vi "Vision Processing.vi"(4 "error in (no error)":errorcluster, 7 "Image Size":T1=enum."320x240") -> ()   [LabVIEW 2015]
doc: "This VI runs in parallel to other tasks. It gets images from the camera, processes them for color or shape and use that information to affect robot behavior."
uses:
  <vilib>/Rock Robotics/WPI/Camera/WPI_CameraImageSize.ctl
  <vilib>/Rock Robotics/WPI/Camera/WPI_CameraWhite Balance Values.ctl
  <vilib>/Rock Robotics/WPI/Camera/WPI_CameraExposure Values.ctl
  <vilib>/Rock Robotics/WPI/Camera/WPI_CameraFrameRate.ctl
  Robot Global Data.vi
panel:
  in  "Image Size 2":T1=enum."320x240"
  in  "error in (no error) 2":errorcluster
  in  "stop":bool
  in  "Target Template":enum32{"Template 3", "Template 1", "Template 2"}(radio)=enum."Template 1"
  out "Input Image":T2(plugin-control)
  out "Processed Image":T2(plugin-control)
  in  "Loop Delay (ms)":u32(slide)=200 scale=0.0..250.0
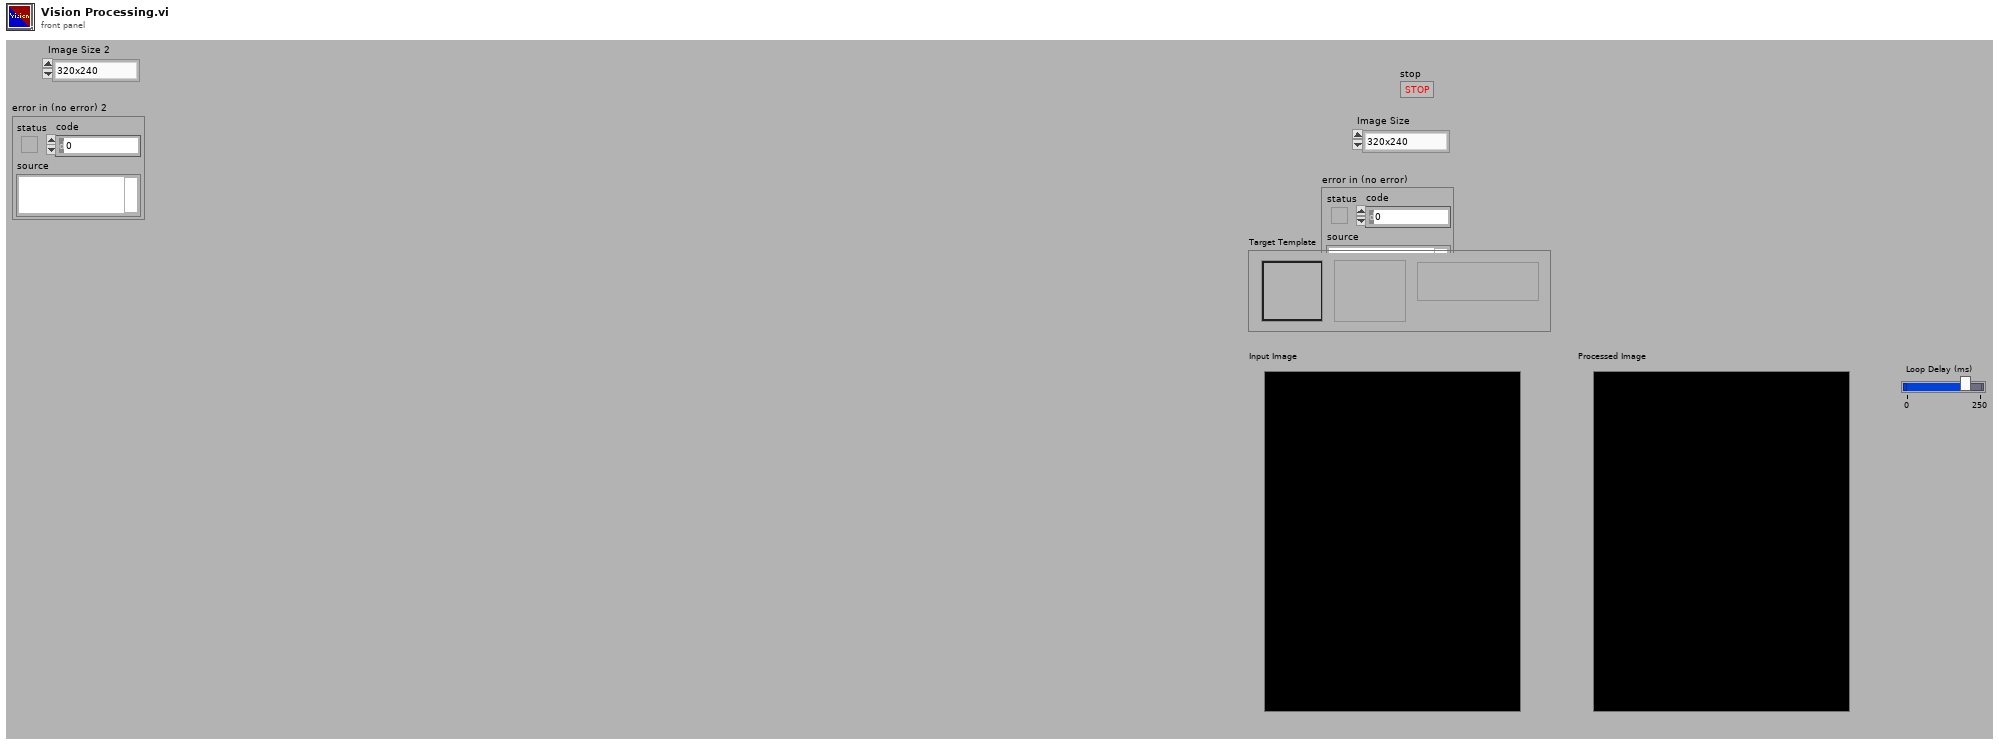
[diagram p1: front panel]
types:
  T1 = typedef "WPI_CameraImageSize.ctl" = enum16{"640x480", "320x240", "160x120", "Custom"}
  T2 = typedef "IMAQ Image.ctl" = refnum<image>
  T3 = typedef "WPI_CameraFrameRate.ctl" = u32
  T4 = typedef "WPI_CameraExposure Values.ctl" = enum16{"Auto", "Flicker-free 50 Hz", "Flicker-free 60 Hz", "Hold current", "Custom"}
  T5 = typedef "WPI_CameraWhite Balance Values.ctl" = enum16{"Auto", "Fixed indoor", "Fixed outdoor 1", "Fixed outdoor 2", "Fixed fluorescent 1", "Fixed fluorescent 2", "Hold current", "Custom"}
  T6 = typedef "Image Type" = u32
  T7 = typedef "WPI_CameraDevRef.ctl" = cluster{"Camera Address":string, "CameraStatus":errorcluster}
  T8 = cluster{"Position":cluster{"x":sgl, "y":sgl}, "Angle":sgl, "Scale":sgl, "Score":sgl, "Bounding Box":cluster{"x":sgl, "y":sgl}[]}[]
  T9 = typedef "ROI Descriptor" = cluster{"Global Rectangle":i32[], "Contours":cluster{"ID":enum32{"External", "Internal"}, "Type":u32, "Coordinates":i32[]}[]}
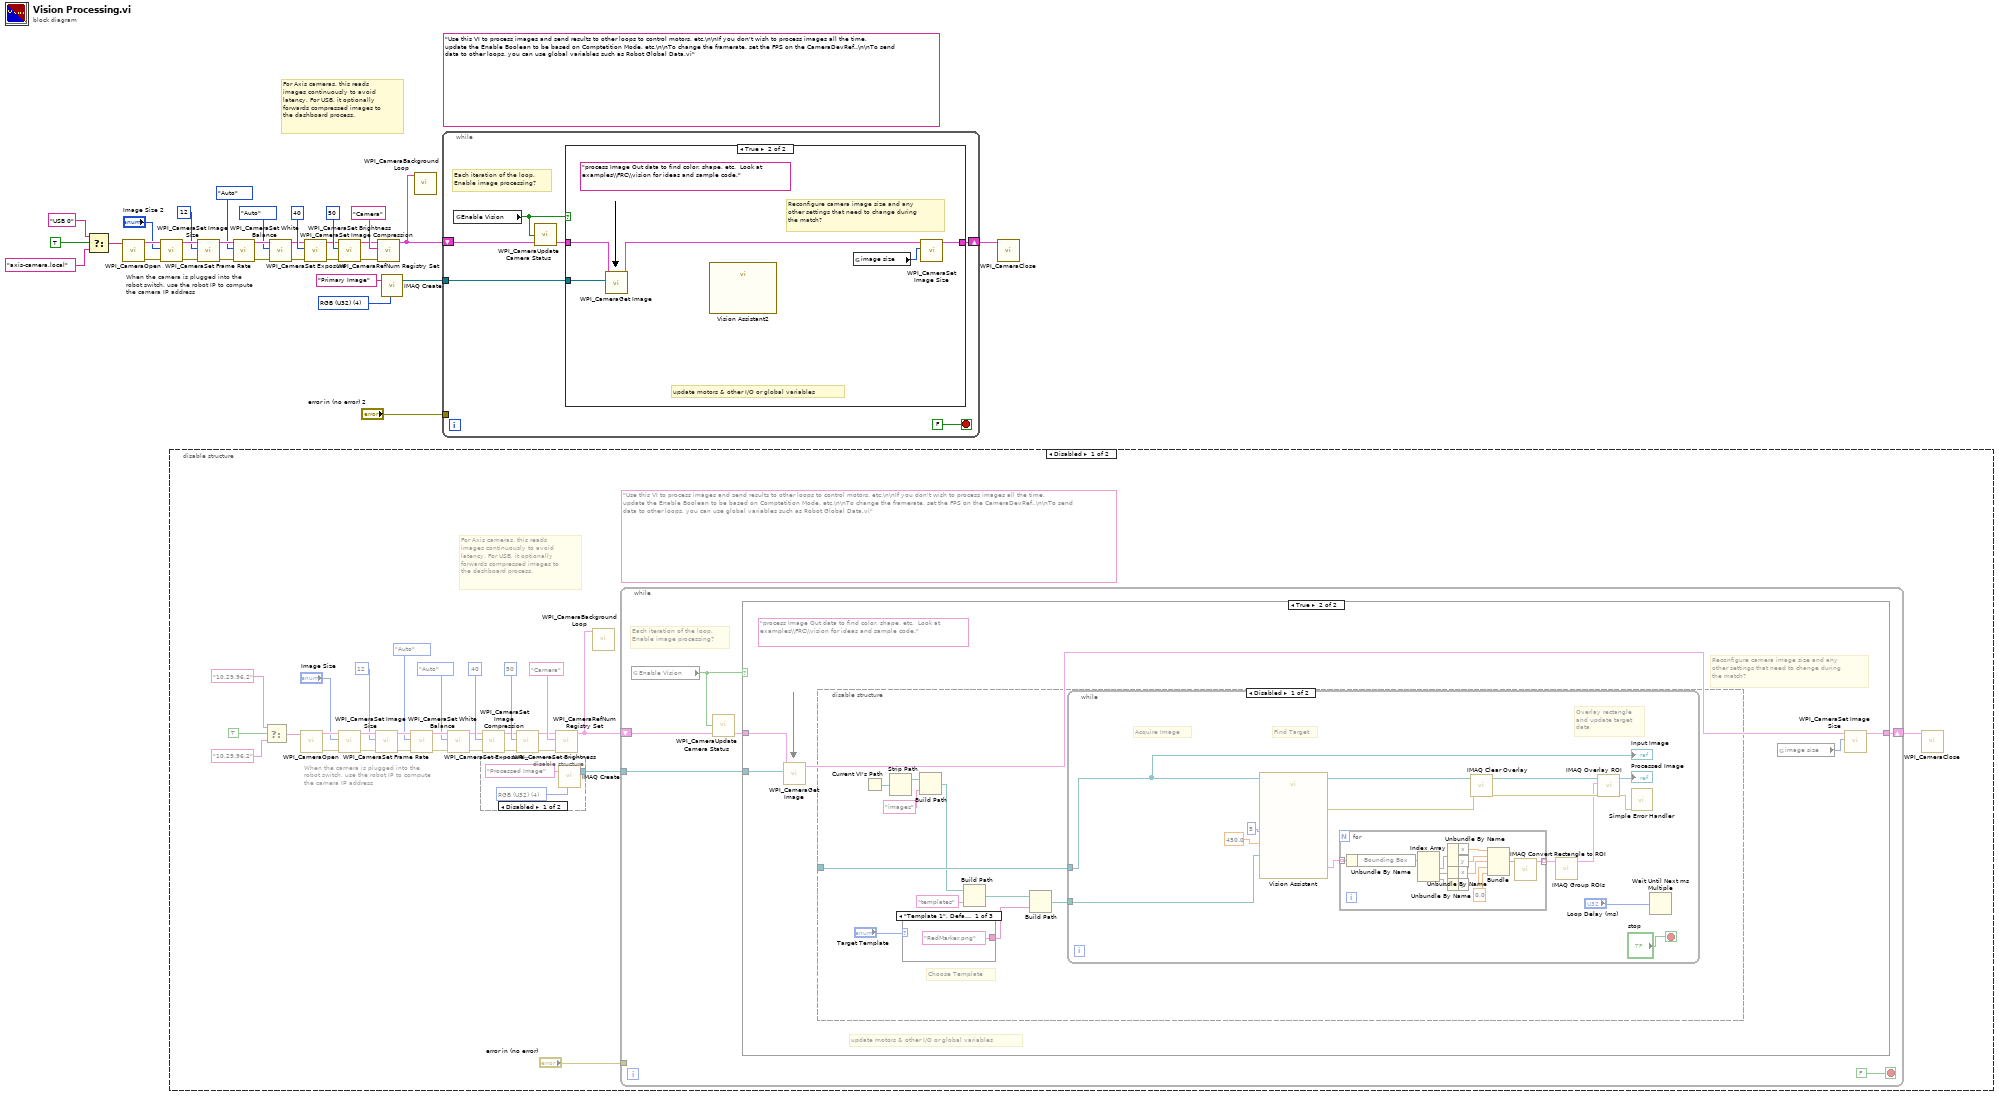
[diagram p0: block diagram]
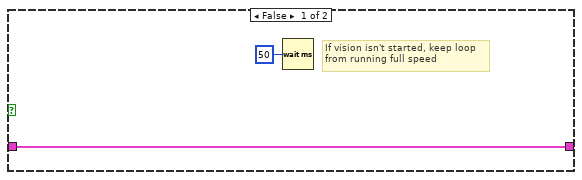
[diagram p2: hidden frame]
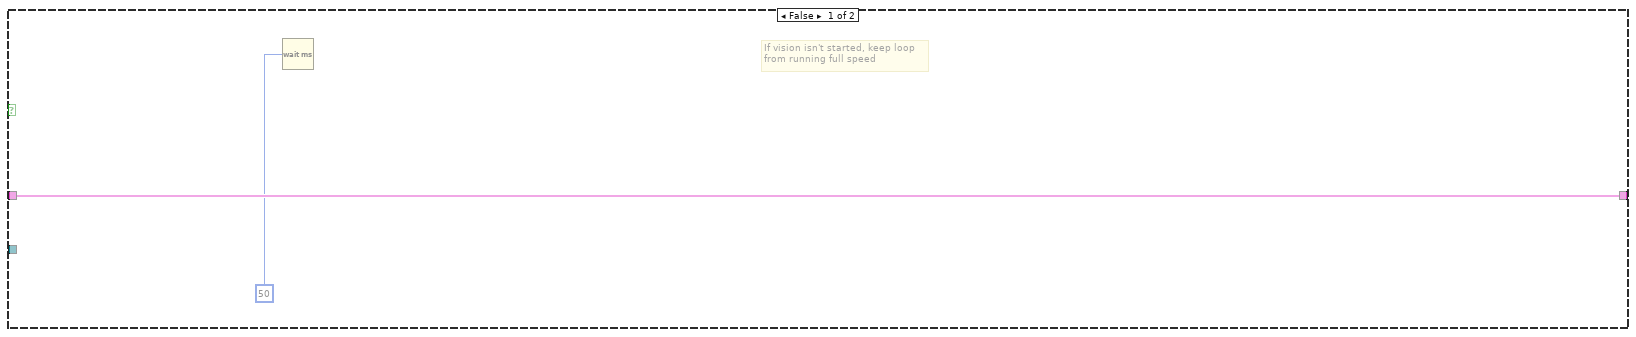
[diagram p4: hidden frame]
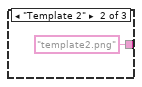
[diagram p5: hidden frame]
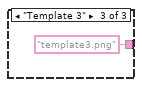
[diagram p6: hidden frame]
diagram:
  (unwired) "Use this VI to process images and send results to other loops to control motors, etc.\n\nIf you don't wish to process images all the time, update the Enable Boolean to be based on Comptetition Mode, etc.\n\nTo change the framerate, set the FPS on the CameraDevRef..\n\nTo send data to other loops, you can use global variables such as Robot Global Data.vi"
  w31 = T6 4 items=["Grayscale (U8)", "Grayscale (I16)", "Grayscale (SGL)", "Complex (CSG)", "RGB (U32)", "HSL (U32)", "RGB (U64)"] ("Image Type")
  # "When the camera is plugged into the\nrobot switch, use the robot IP to compute\nthe camera IP address"
  # "For Axis cameras, this reads\nimages continuously to avoid\nlatency. For USB, it optionally\nforwards compressed images to\nthe dashboard process."
  n1 = Select(t="USB 0" ("format string"), s=TRUE ("dot notation? (F)"), f="axis-camera.local" ("format string")) -> (s? t:f=w2:string)
  n2 = call <vilib>:"WPI_CameraOpen.vi"("Camera Address"=w2) -> ("error out"=w19:errorcluster, "CameraDevRef"=w20:T7)  [unwired: 1 in, 8 out]
  n3 = call <vilib>:"WPI_CameraSet Image Size.vi"("error in (no error)"=w19, "Image Size"="Image Size 2", "CameraDevRef"=w20) -> ("error out"=w18:errorcluster, "CameraDevRef Out"=w21:T7)  [unwired: 1 in, 6 out]
  n4 = disable-structure shown="Disabled" {
    frame Disabled {
      (unwired) "Use this VI to process images and send results to other loops to control motors, etc.\n\nIf you don't wish to process images all the time, update the Enable Boolean to be based on Comptetition Mode, etc.\n\nTo change the framerate, set the FPS on the CameraDevRef..\n\nTo send data to other loops, you can use global variables such as Robot Global Data.vi"
      # "When the camera is plugged into the\nrobot switch, use the robot IP to compute\nthe camera IP address"
      # "For Axis cameras, this reads\nimages continuously to avoid\nlatency. For USB, it optionally\nforwards compressed images to\nthe dashboard process."
      n5 = Select(t="10.29.96.2" ("format string"), s=TRUE ("dot notation? (F)"), f="10.29.96.2" ("format string")) -> (s? t:f=w33:string)
      n6 = call <vilib>:"WPI_CameraOpen.vi"("Camera Address"=w33) -> ("error out"=w50:errorcluster, "CameraDevRef"=w51:T7)  [unwired: 1 in, 8 out]
      n7 = call <vilib>:"WPI_CameraSet Image Size.vi"("error in (no error)"=w50, "Image Size"="Image Size", "CameraDevRef"=w51) -> ("error out"=w49:errorcluster, "CameraDevRef Out"=w52:T7)  [unwired: 1 in, 6 out]
      n8 = call <vilib>:"WPI_CameraSet Frame Rate.vi"("error in (no error)"=w49, "Frame Rate (fps)"=T3 12, "CameraDevRef"=w52) -> ("error out"=w48:errorcluster, "CameraDevRef Out"=w54:T7)  [unwired: 7 out]
      n9 = call <vilib>:"WPI_CameraSet White Balance.vi"("error in (no error)"=w48, "White Balance"=WPI_CameraWhite_Balance_Values."Auto", "CameraDevRef"=w54) -> ("error out"=w47:errorcluster, "CameraDevRef Out"=w53:T7)  [unwired: 1 in, 6 out]
      n10 = call <vilib>:"WPI_CameraSet Exposure.vi"("error in (no error)"=w47, "Exposure"=WPI_CameraExposure_Values."Auto", "CameraDevRef"=w53) -> ("error out"=w46:errorcluster, "CameraDevRef Out"=w56:T7)  [unwired: 1 in, 6 out]
      n11 = disable-structure shown="Disabled" {
        disable-tunnel: [w61 _] -> w60
        frame Disabled {
          w63 = T6 4 items=["Grayscale (U8)", "Grayscale (I16)", "Grayscale (SGL)", "Complex (CSG)", "RGB (U32)", "HSL (U32)", "RGB (U64)"] ("Image Type")
          n12 = call "IMAQ Create"("Image Name"="Processed Image", "Image Type"=w63) -> ("New Image"=w61:T2)  [unwired: 2 in, 2 out]
        }
        frame Enabled {
        }
      }
      n13 = call <vilib>:"WPI_CameraSet Image Compression.vi"("error in (no error)"=w46, "Compression"=40, "CameraDevRef"=w56) -> ("error out"=w45:errorcluster, "CameraDevRef Out"=w55:T7)  [unwired: 7 out]
      n14 = call <vilib>:"WPI_CameraSet Brightness.vi"("error in (no error)"=w45, "Brightness"=50, "CameraDevRef"=w55) -> ("error out"=w43:errorcluster, "CameraDevRef Out"=w44:T7)  [unwired: 7 out]
      n15 = call <vilib>:"WPI_CameraRefNum Registry Set.vi"("error in (no error)"=w43, "refnum name"="Camera", "CameraDevRef"=w44) -> ("CameraDevRef"=w39:T7)  [unwired: 1 in, 7 out]
      n16 = call <vilib>:"WPI_CameraBackground Loop.vi"("CameraDevRef"=w39) -> ()  [unwired: 11 in]
      n17 = while {
        shift-right: [w68] -> w37
        shift-left: w39 -> [w66]
        tunnel: w60 -> [w67]
        tunnel: "error in (no error)" -> [_]
        stop <- FALSE stop-if-true
        # "Each iteration of the loop,\nEnable image processing?"
        n18 = global read "Robot Global Data.vi" "Enable Vision"() -> (w64:bool)
        n19 = call <vilib>:"WPI_CameraUpdate Camera Status.vi"("CameraDevRef In"=w66, "Enable Vision"=w64) -> ("CameraDevRef Out"=w65:T7)  [unwired: 3 in]
        n20 = case shown="True" w64 {
          tunnel: w67 -> [_ w75]
          tunnel: [w71 w76] -> w68
          tunnel: w65 -> [w71 w73]
          frame False {
            # "If vision isn't started, keep loop\nfrom running full speed"
            n21 = Wait (ms)(milliseconds to wait=u32 50) -> ()  [unwired: 1 out]
          }
          frame True {
            (unwired) "process Image Out data to find color, shape, etc.  Look at examples\\FRC\\vision for ideas and sample code."
            # "update motors & other I/O or global variables"
            # "Reconfigure camera image size and any\nother settings that need to change during\nthe match?"
            n22 = call <vilib>:"WPI_CameraGet Image.vi"("Image"=w75, "CameraDevRef"=w73) -> ("CameraDevRef Out"=w72:T7)  [unwired: 1 in, 8 out]
            n23 = disable-structure shown="Disabled" {
              disable-tunnel: _ -> [w86 _]
              frame Disabled {
                # "Choose Template"
                n24 = Current VI's Path() -> (path=w85:path)
                n25 = Strip Path(path=w85) -> (stripped path=w80:path)  [unwired: 1 out]
                n26 = case shown="\"Template 1\", Default" "Target Template" {
                  tunnel: ["RedMarker.png" ("name or relative path") "template2.png" ("name or relative path") "template3.png" ("name or relative path")] -> w81
                  frame "Template 1", Default {
                  }
                  frame "Template 2" {
                  }
                  frame "Template 3" {
                  }
                }
                n27 = Build Path(base path=w80, name or relative path="images") -> (appended path=w78:path)
                n28 = Build Path(base path=w78, name or relative path="templates") -> (appended path=w77:path)
                n29 = Build Path(base path=w77, name or relative path=w81) -> (appended path=w83:path)
                n30 = while {
                  tunnel: w83 -> [w92]
                  tunnel: w86 -> [w90]
                  stop <- "stop" stop-if-true
                  # "Overlay rectangle\nand update target\ndata"
                  # "Find Target"
                  # "Acquire Image"
                  n31 = call "Vision Assistant"("Image In"=w90, "Number of Matches Requested (Pattern Matching)"=5 ("Number of Matches Requested (Pattern Matching 1)"), "Minimum Match Score (Pattern Matching)"=sgl 450.0 ("Minimum Match Score"), "Template File Path (Pattern Matching)"=w92) -> ("Image Out"=w104:T2, "Matches (Pattern Matching)"=w96:T8, "error out"=w102:errorcluster)  [unwired: 2 in, 19 out]
                  n32 = for {
                    tunnel: w96 -> [w116] mode=indexing
                    tunnel: [w107] -> w95 mode=indexing
                    n33 = Unbundle By Name(w116) -> ("Bounding Box"=w115:cluster{"x":sgl, "y":sgl}[])
                    n34 = Index Array(array=w115) -> (element #1=w114:cluster{"x":sgl, "y":sgl}, element #2=w113:cluster{"x":sgl, "y":sgl}, element #3=w106:cluster{"x":sgl, "y":sgl})  [unwired: 3 in]
                    n35 = Unbundle By Name(w114) -> ("x"=w112:sgl, "y"=w111:sgl)
                    n36 = Unbundle By Name(w113) -> ("x"=w110:sgl)
                    n37 = Unbundle By Name(w106) -> ("y"=w105:sgl)
                    n38 = Bundle("x"=w112, "y"=w111, "x"=w110, "y"=w105, 0.0) -> (w108:cluster{"x":sgl, "y":sgl, "x":sgl, "y":sgl, dbl})  [unwired: 1 out]
                    n39 = call "IMAQ Convert Rectangle to ROI"("Rectangle"=w108) -> ("ROI Descriptor"=w107:T9)  [unwired: 1 in, 8 out]
                  }
                  n40 = call "IMAQ Clear Overlay"("error in (no error)"=w102, "Image"=w104) -> ("error out"=w101:errorcluster, "Image Out"=w93:T2)  [unwired: 1 in, 7 out]
                  n41 = call "IMAQ Group ROIs"("ROI Descriptors"=w95) -> ("ROI Descriptor out"=w94:T9)  [unwired: 1 in, 3 out]
                  n42 = call "IMAQ Overlay ROI"("error in (no error)"=w101, "ROI Descriptor"=w94, "Image"=w93) -> ("error out"=w99:errorcluster, "Image Out"=→"Processed Image":T2)  [unwired: 3 in, 4 out]
                  n43 = call <vilib>:"Simple Error Handler.vi"("error in (no error)"=w99) -> ()  [unwired: 1 in, 8 out]
                  n44 = Wait Until Next ms Multiple(millisecond multiple="Loop Delay (ms)") -> ()  [unwired: 1 out]
                  "Input Image" <- w90
                }
              }
              frame Enabled {
              }
            }
            n45 = global read "Robot Global Data.vi" "image size"() -> (w74:T1)
            n46 = call <vilib>:"WPI_CameraSet Image Size.vi"("Image Size"=w74, "CameraDevRef"=w72) -> ("CameraDevRef Out"=w76:T7)  [unwired: 2 in, 7 out]
          }
        }
      }
      n47 = call <vilib>:"WPI_CameraClose.vi"("CameraDevRef"=w37) -> ()  [unwired: 1 in, 10 out]
    }
    frame Enabled {
    }
  }
  n48 = call <vilib>:"WPI_CameraSet Frame Rate.vi"("error in (no error)"=w18, "Frame Rate (fps)"=T3 12, "CameraDevRef"=w21) -> ("error out"=w17:errorcluster, "CameraDevRef Out"=w23:T7)  [unwired: 7 out]
  n49 = call <vilib>:"WPI_CameraSet White Balance.vi"("error in (no error)"=w17, "White Balance"=WPI_CameraWhite_Balance_Values."Auto", "CameraDevRef"=w23) -> ("error out"=w16:errorcluster, "CameraDevRef Out"=w22:T7)  [unwired: 1 in, 6 out]
  n50 = call <vilib>:"WPI_CameraSet Exposure.vi"("error in (no error)"=w16, "Exposure"=WPI_CameraExposure_Values."Auto", "CameraDevRef"=w22) -> ("error out"=w15:errorcluster, "CameraDevRef Out"=w25:T7)  [unwired: 1 in, 6 out]
  n51 = call <vilib>:"WPI_CameraSet Image Compression.vi"("error in (no error)"=w15, "Compression"=40, "CameraDevRef"=w25) -> ("error out"=w14:errorcluster, "CameraDevRef Out"=w24:T7)  [unwired: 7 out]
  n52 = call <vilib>:"WPI_CameraSet Brightness.vi"("error in (no error)"=w14, "Brightness"=50, "CameraDevRef"=w24) -> ("error out"=w12:errorcluster, "CameraDevRef Out"=w13:T7)  [unwired: 7 out]
  n53 = call <vilib>:"WPI_CameraRefNum Registry Set.vi"("error in (no error)"=w12, "refnum name"="Camera", "CameraDevRef"=w13) -> ("CameraDevRef"=w8:T7)  [unwired: 1 in, 7 out]
  n54 = call "IMAQ Create"("Image Name"="Primary Image", "Image Type"=w31) -> ("New Image"=w29:T2)  [unwired: 2 in, 2 out]
  n55 = call <vilib>:"WPI_CameraBackground Loop.vi"("CameraDevRef"=w8) -> ()  [unwired: 11 in]
  n56 = while {
    shift-right: [w121] -> w6
    shift-left: w8 -> [w119]
    tunnel: w29 -> [w120]
    tunnel: "error in (no error) 2" -> [_]
    stop <- FALSE stop-if-true
    # "Each iteration of the loop,\nEnable image processing?"
    n57 = global read "Robot Global Data.vi" "Enable Vision"() -> (w117:bool)
    n58 = call <vilib>:"WPI_CameraUpdate Camera Status.vi"("CameraDevRef In"=w119, "Enable Vision"=w117) -> ("CameraDevRef Out"=w118:T7)  [unwired: 3 in]
    n59 = case shown="True" w117 {
      tunnel: w120 -> [_ w128]
      tunnel: [w124 w129] -> w121
      tunnel: w118 -> [w124 w126]
      frame False {
        # "If vision isn't started, keep loop\nfrom running full speed"
        n60 = Wait (ms)(milliseconds to wait=u32 50) -> ()  [unwired: 1 out]
      }
      frame True {
        (unwired) "process Image Out data to find color, shape, etc.  Look at examples\\FRC\\vision for ideas and sample code."
        # "update motors & other I/O or global variables"
        # "Reconfigure camera image size and any\nother settings that need to change during\nthe match?"
        n61 = call <vilib>:"WPI_CameraGet Image.vi"("Image"=w128, "CameraDevRef"=w126) -> ("CameraDevRef Out"=w125:T7)  [unwired: 1 in, 8 out]
        n62 = call "Vision Assistant2"() -> ()  [unwired: 12 in]
        n63 = global read "Robot Global Data.vi" "image size"() -> (w127:T1)
        n64 = call <vilib>:"WPI_CameraSet Image Size.vi"("Image Size"=w127, "CameraDevRef"=w125) -> ("CameraDevRef Out"=w129:T7)  [unwired: 2 in, 7 out]
      }
    }
  }
  n65 = call <vilib>:"WPI_CameraClose.vi"("CameraDevRef"=w6) -> ()  [unwired: 1 in, 10 out]
